vi "Read XtraJsonEncodeObj.vi"(8 "error in (no error)":errorcluster, 11 "LogMap in":refnum<class "LogMap.lvclass">) -> (0 "error out":errorcluster, 2 "XtraJsonEncodeObj":bool, 3 "LogMap out":refnum<class "LogMap.lvclass">)   [LabVIEW 2020, in "ORM.lvlib" / "LogMap.lvclass"]
uses:
  LogMap.lvclass
  LogMap.lvclass/LogMap.ctl
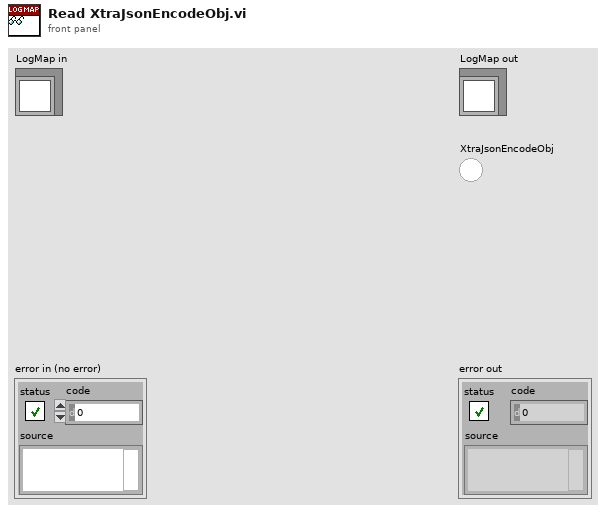
[diagram p1: front panel]
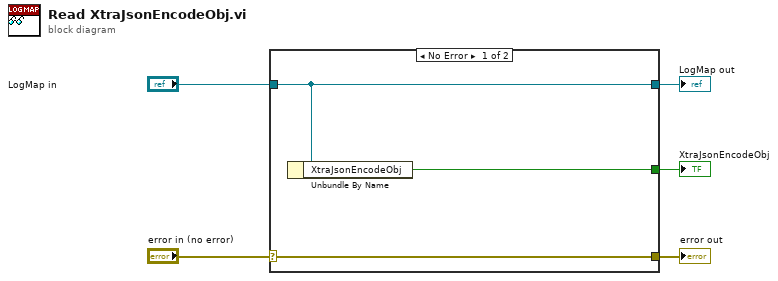
[diagram p0: block diagram]
diagram:
  n1 = case shown="No Error" "error in (no error)" {
    selector: "error in (no error)" -> [w8 w9]
    tunnel: [w8 w9] -> w4
    tunnel: [w7 w10] -> w2
    tunnel: "LogMap in" -> [w7 w10]
    tunnel: [w6 _] -> w1
    frame No Error {
      n2 = Unbundle By Name(w7) -> ("XtraJsonEncodeObj"=w6:bool)
    }
    frame Error {
    }
  }
  "error out" <- w4
  "LogMap out" <- w2
  "XtraJsonEncodeObj" <- w1
